vi "DAQNavi Read (Analog 1D DBL NChan 1Samp).vi"(8 "error in (no error)":errorcluster, 10 "timeout":dbl=10.0 format="%0.2f", 11 "task in":i32) -> (0 "error out":errorcluster, 2 "data":dbl[](array[numeric]), 3 "task out":i32)   [LabVIEW 2020]
uses:
  DAQNavi_LV.dll
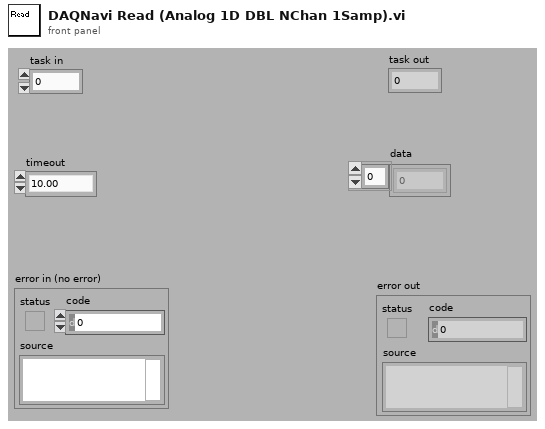
[diagram p1: front panel]
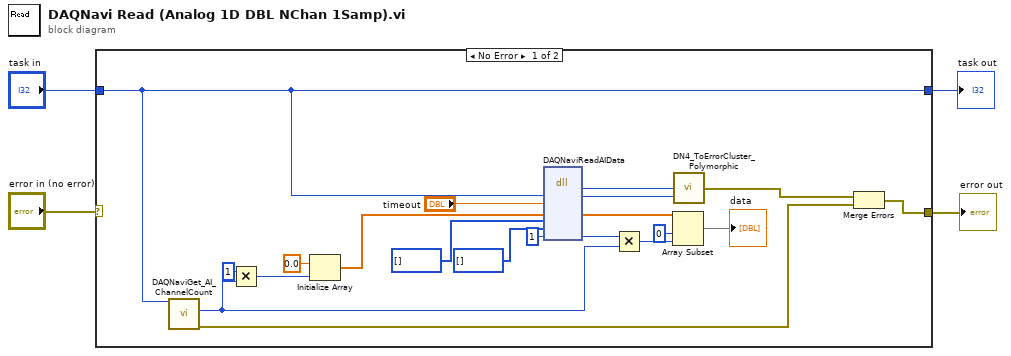
[diagram p0: block diagram]
diagram:
  n1 = case shown="No Error" "error in (no error)" {
    selector: "error in (no error)" -> [_ w25]
    tunnel: "task in" -> [w16 w26]
    tunnel: [w16 w26] -> w2
    tunnel: [w13 w25] -> w1
    frame No Error {
      n2 = call "DAQNaviGet_AI_ChannelCount.vi"("task in"=w16) -> ("error out"=w14:errorcluster, "channel count"=w7:i32)  [unwired: 1 in, 8 out]
      n3 = Multiply(x=1 ("y"), y=w7) -> (x*y=w17:i32)
      n4 = Initialize Array(0.0 ("element"), w17) -> (w10:dbl[])
      n5 = dll-call lib="DAQNavi_LV.dll" fn="DAQNaviReadAIData"("taskID"=w16, "timeout"="timeout", "scaledData"=w10, "rawData16"=u16[] [] ("scaledData"), "rawData32"=u32[] [], "samples"=1) -> ("return type"=w20:i32, "taskID"=w5:i32, "scaledData"=w9:dbl[], "samples"=w8:i32)  [unwired: 4 in, 4 out]
      n6 = Multiply(x=w8, y=w7) -> (x*y=w6:i32)
      n7 = Array Subset(array=w9, index=0, length=w6) -> (→"data":dbl[])
      n8 = call "DN4_ToErrorCluster_Polymorphic.vi"("task id"=w5, "error code"=w20) -> ("error out"=w15:errorcluster)  [unwired: 3 out]
      n9 = Merge Errors(w15, w14) -> (w13:errorcluster)
    }
    frame Error {
    }
  }
  "task out" <- w2
  "error out" <- w1
